vi "Configure DC Current4.vi"(8 "error in (no error)":errorcluster, 10 "measurementservice_SMUConfigRequest_Data":T1) -> (0 "error out":errorcluster, 2 "measurementservice_SMUConfigRequest_Data Out":T1)   [LabVIEW 2019, in "HVC4.lvlib" / "HVC4.lvclass"]
doc: "Demonstrates how to use the DC Current Output Function to force an output current. This example initializes a session, configures the Output Function, Sense, Autorange, Current Level and Voltage Limit, initiates generation, waits for a specified delay, and measures the voltage and current output. This example uses Single Point source mode."
uses:
  HVC4 Class/HVC4.lvclass
  HVC4 Class/RPC Messages/measurementservice_SMUConfigRequest/measurementservice_SMUConfigRequest_Data.ctl
panel:
  # "Overview: Demonstrates how to use the DC Current Output Function to force an output current.  \nThis example initializes a session, configures the Output Function, Sense, Autorange, Current Level \nand Voltage Limit, initiates generation, waits for a specified delay, and measures the voltage and \ncurrent output.  \nRequirements: NI-DCPower\nInstructions:\n1. Select the appropriate device in the Resource Name control.\n2. Configure the parameters of the DC Current signal you'd like to output.\n3. Run the VI."
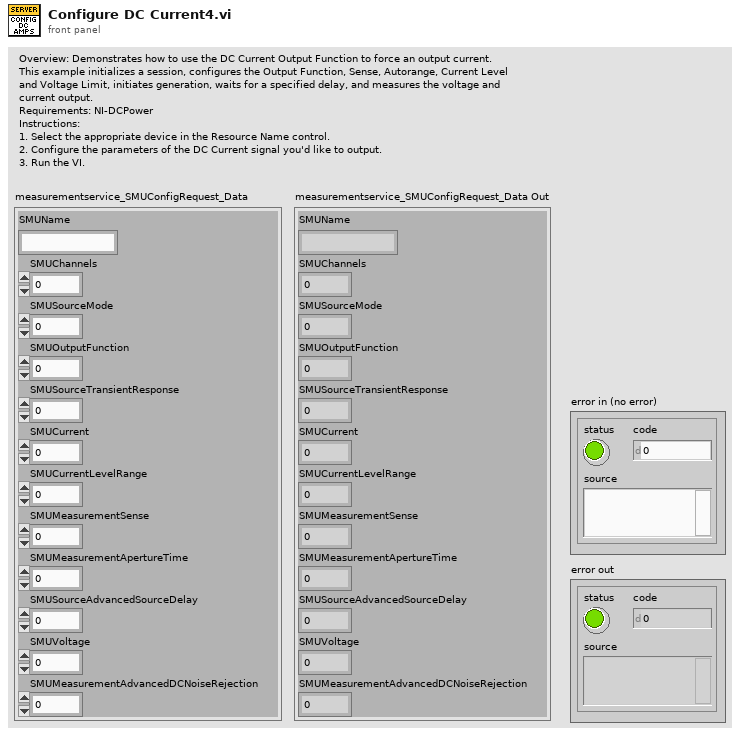
[diagram p1: front panel]
types:
  T1 = typedef "HVC4.lvlib/HVC4.lvclass/measurementservice_SMUConfigRequest_Data.ctl" = cluster{"SMUName":string, "SMUChannels":i32, "SMUSourceMode":i32, "SMUOutputFunction":i32, "SMUSourceTransientResponse":i32, "SMUCurrent":sgl, "SMUCurrentLevelRange":sgl, "SMUMeasurementSense":i32, "SMUMeasurementApertureTime":sgl, "SMUSourceAdvancedSourceDelay":sgl, "SMUVoltage":sgl, "SMUMeasurementAdvancedDCNoiseRejection":i32}
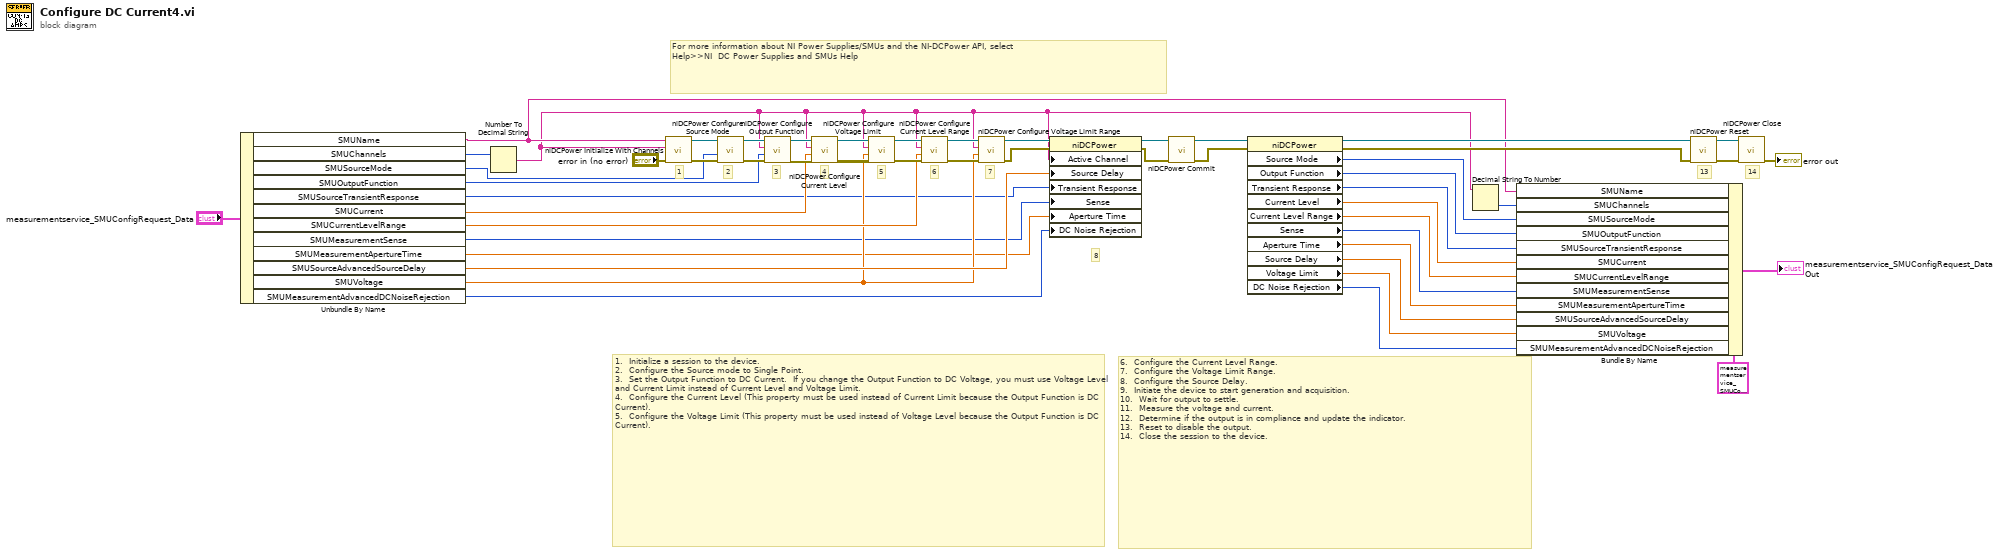
[diagram p0: block diagram]
diagram:
  # "For more information about NI Power Supplies/SMUs and the NI-DCPower API, select\nHelp>>NI  DC Power Supplies and SMUs Help"
  # "14"
  # "8"
  # "7"
  # "6"
  # "2"
  # "1.  Initialize a session to the device.\n2.  Configure the Source mode to Single Point.\n3.  Set the Output Function to DC Current.  If you change the Output Function to DC Voltage, you must use Voltage Level and Current Limit instead of Current Level and Voltage Limit.\n4.  Configure the Current Level (This property must be used instead of Current Limit because the Output Function is DC Current).\n5.  Configure the Voltage Limit (This property must be used instead of Voltage Level because the Output Function is DC Current)."
  # "3"
  # "6.  Configure the Current Level Range.\n7.  Configure the Voltage Limit Range.\n8.  Configure the Source Delay.\n9.  Initiate the device to start generation and acquisition.\n10.  Wait for output to settle.\n11.  Measure the voltage and current.\n12.  Determine if the output is in compliance and update the indicator.\n13.  Reset to disable the output.\n14.  Close the session to the device."
  # "13"
  # "5"
  # "4"
  # "1"
  n1 = Unbundle By Name("measurementservice_SMUConfigRequest_Data") -> ("SMUName"=w14:string, "SMUChannels"=w28:i32, "SMUSourceMode"=w27:i32, "SMUOutputFunction"=w26:i32, "SMUSourceTransientResponse"=w21:i32, "SMUCurrent"=w25:sgl, "SMUCurrentLevelRange"=w24:sgl, "SMUMeasurementSense"=w20:i32, "SMUMeasurementApertureTime"=w19:sgl, "SMUSourceAdvancedSourceDelay"=w23:sgl, "SMUVoltage"=w22:sgl, "SMUMeasurementAdvancedDCNoiseRejection"=w18:i32)
  n2 = Number To Decimal String(number=w28) -> (decimal integer string=w12:string)  [unwired: 1 in]
  n3 = call <instrlib>:"niDCPower Initialize With Channels.vi"("error in (no error)"="error in (no error)", "channels"=w12, "resource name"=w14) -> ("error out"=w45:errorcluster, "instrument handle out"=w44:refnum<k15>)  [unwired: 2 in, 5 out]
  n4 = call <instrlib>:"niDCPower Configure Source Mode.vi"("error in (no error)"=w45, "source mode"=w27, "instrument handle"=w44) -> ("error out"=w43:errorcluster, "instrument handle out"=w42:refnum<k15>)  [unwired: 7 out]
  n5 = call <instrlib>:"niDCPower Configure Output Function.vi"("error in (no error)"=w43, "output function"=w26, "channel name"=w12, "instrument handle"=w42) -> ("error out"=w35:errorcluster, "instrument handle out"=w34:refnum<k15>)  [unwired: 6 out]
  n6 = call <instrlib>:"niDCPower Configure Current Level.vi"("error in (no error)"=w35, "current level"=w25, "channel name"=w12, "instrument handle"=w34) -> ("error out"=w49:errorcluster, "instrument handle out"=w50:refnum<k15>)  [unwired: 6 out]
  n7 = call <instrlib>:"niDCPower Configure Voltage Limit.vi"("error in (no error)"=w49, "voltage limit"=w22, "channel name"=w12, "instrument handle"=w50) -> ("error out"=w41:errorcluster, "instrument handle out"=w40:refnum<k15>)  [unwired: 6 out]
  n8 = call <instrlib>:"niDCPower Configure Current Level Range.vi"("error in (no error)"=w41, "current level range"=w24, "channel name"=w12, "instrument handle"=w40) -> ("error out"=w39:errorcluster, "instrument handle out"=w38:refnum<k15>)  [unwired: 6 out]
  n9 = call <instrlib>:"niDCPower Configure Voltage Limit Range.vi"("error in (no error)"=w39, "voltage limit range"=w22, "channel name"=w12, "instrument handle"=w38) -> ("error out"=w36:errorcluster, "instrument handle out"=w37:refnum<k15>)  [unwired: 6 out]
  n10 = property class="niDCPower"(reference=w37, error in=w36, "Active Channel"=w12, "Source Delay"=w23, "Transient Response"=w21, "Sense"=w20, "Aperture Time"=w19, "DC Noise Rejection"=w18) -> (reference out=w33:refnum<k15>, error out=w32:errorcluster)
  n11 = call <instrlib>:"niDCPower Commit.vi"("error in (no error)"=w32, "instrument handle"=w33) -> ("error out"=w30:errorcluster, "instrument handle out"=w31:refnum<k15>)  [unwired: 8 in]
  n12 = property class="niDCPower"(reference=w31, error in=w30) -> (error out=w29:errorcluster, "Source Mode"=w11:i32, "Output Function"=w10:i32, "Transient Response"=w9:i32, "Current Level"=w8:dbl, "Current Level Range"=w7:dbl, "Sense"=w6:i32, "Aperture Time"=w5:dbl, "Source Delay"=w4:dbl, "Voltage Limit"=w3:dbl, "DC Noise Rejection"=w2:i32)  [unwired: 1 out]
  n13 = Decimal String To Number(string=w12) -> (number=w13:i32)  [unwired: 2 in, 1 out]
  n14 = Bundle By Name(cluster=T1 {"SMUName"="", "SMUChannels"=0, "SMUSourceMode"=0, "SMUOutputFunction"=0, "SMUSourceTransientResponse"=0, "SMUCurrent"=0.0, "SMUCurrentLevelRange"=0.0, "SMUMeasurementSense"=0, "SMUMeasurementApertureTime"=0.0, "SMUSourceAdvancedSourceDelay"=0.0, "SMUVoltage"=0.0, "SMUMeasurementAdvancedDCNoiseRejection"=0} ("measurementservice_SMUConfigRequest_Data Out"), "SMUName"=w14, "SMUChannels"=w13, "SMUSourceMode"=w11, "SMUOutputFunction"=w10, "SMUSourceTransientResponse"=w9, "SMUCurrent"=w8, "SMUCurrentLevelRange"=w7, "SMUMeasurementSense"=w6, "SMUMeasurementApertureTime"=w5, "SMUSourceAdvancedSourceDelay"=w4, "SMUVoltage"=w3, "SMUMeasurementAdvancedDCNoiseRejection"=w2) -> (→"measurementservice_SMUConfigRequest_Data Out":T1)
  n15 = call <instrlib>:"niDCPower Reset.vi"("error in (no error)"=w29, "instrument handle"=w31) -> ("error out"=w47:errorcluster, "instrument handle out"=w48:refnum<k15>)  [unwired: 2 in, 6 out]
  n16 = call <instrlib>:"niDCPower Close.vi"("error in (no error)"=w47, "instrument handle"=w48) -> ("error out"=→"error out":errorcluster)  [unwired: 9 out]
